vi "obwiednia_DimScreen.vi"() -> ()   [LabVIEW 2012]
uses:
  <vilib>/Analysis/3filter.llb/FIR Filter (DBL).vi
  <vilib>/Analysis/baseanly.llb/Mean (DBL).vi
  <vilib>/addons/Sound and Vibration/Order Analysis/Fault Analysis/SVPO Envelope Detection (1 Ch DBL Array).vi
  <vilib>/Utility/file.llb/Read From Spreadsheet File (DBL).vi
  <vilib>/Utility/file.llb/Write To Spreadsheet File (DBL).vi
  <vilib>/Analysis/4window.llb/Hamming Window (DBL).vi
  <vilib>/Analysis/NI_AALBase.lvlib
  <vilib>/Analysis/NI_AALPro.lvlib
  <vilib>/Analysis/NI_AAL_SigProc.lvlib
  <vilib>/addons/Sound and Vibration/Order Analysis/Fault Analysis/SoundVib_FaultAnalysis.lvlib
  <vilib>/gmath/NI_Gmath.lvlib
  user32.dll
panel:
  out "Maks. indeks":i32
  out "Największy wsp.":dbl
  out "Współczynniki":dbl[](array[numeric])
  out "Odległość":dbl[](array[numeric])
  out "Waveform Graph 3":dbl[](graph)
  in  "Liczenie":bool
  in  "Pomiar":bool
  in  "stop":bool
  out "Signal energy":dbl
  out "Frames":dbl[][](array[numeric])
  out "Przekroczenie progu":bool
  out "Tablica ramek":dbl[](graph)
  out "number of columns":i32
  out "number of rows":i32
  out "Threshold Energy":dbl
  out "Diagram energii":dbl[](graph)
  out "size(s)":i32
  out "sum":dbl
  out "Length":dbl
  out "\"Wygładzona\" energia":dbl[](graph)
  out "max index":dbl
  out "min index":dbl
  out "Wypowiedź":dbl[](graph)
  out "Mowa":waveform(dbl)[](graph)
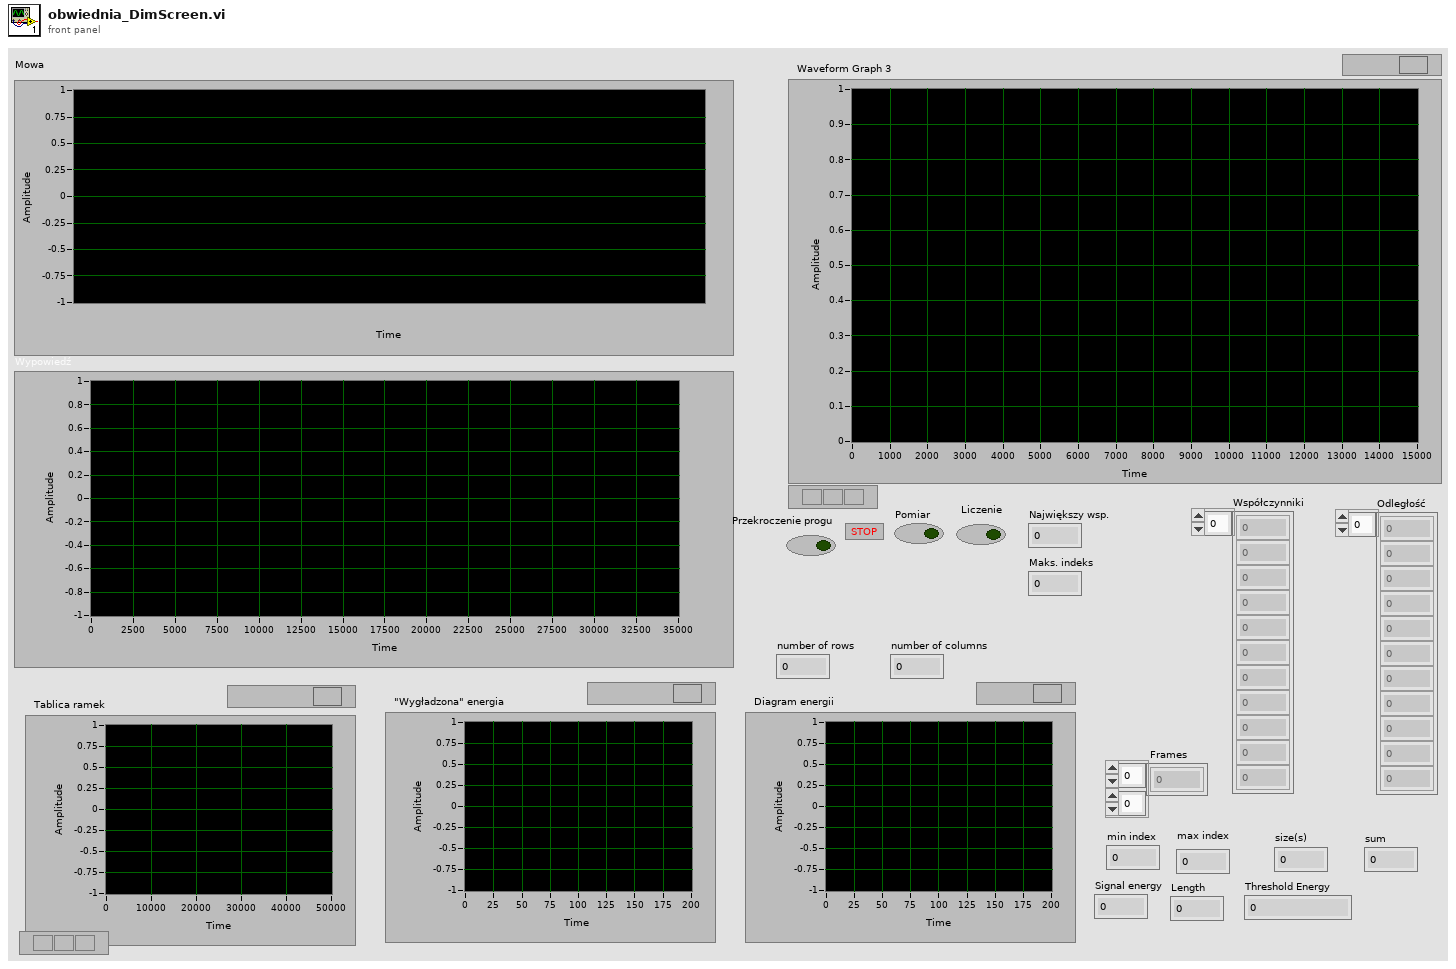
[diagram p1: front panel]
types:
  T1 = enum16{"open", "replace", "create", "open or create", "replace or create", "replace or create with confirmation"}
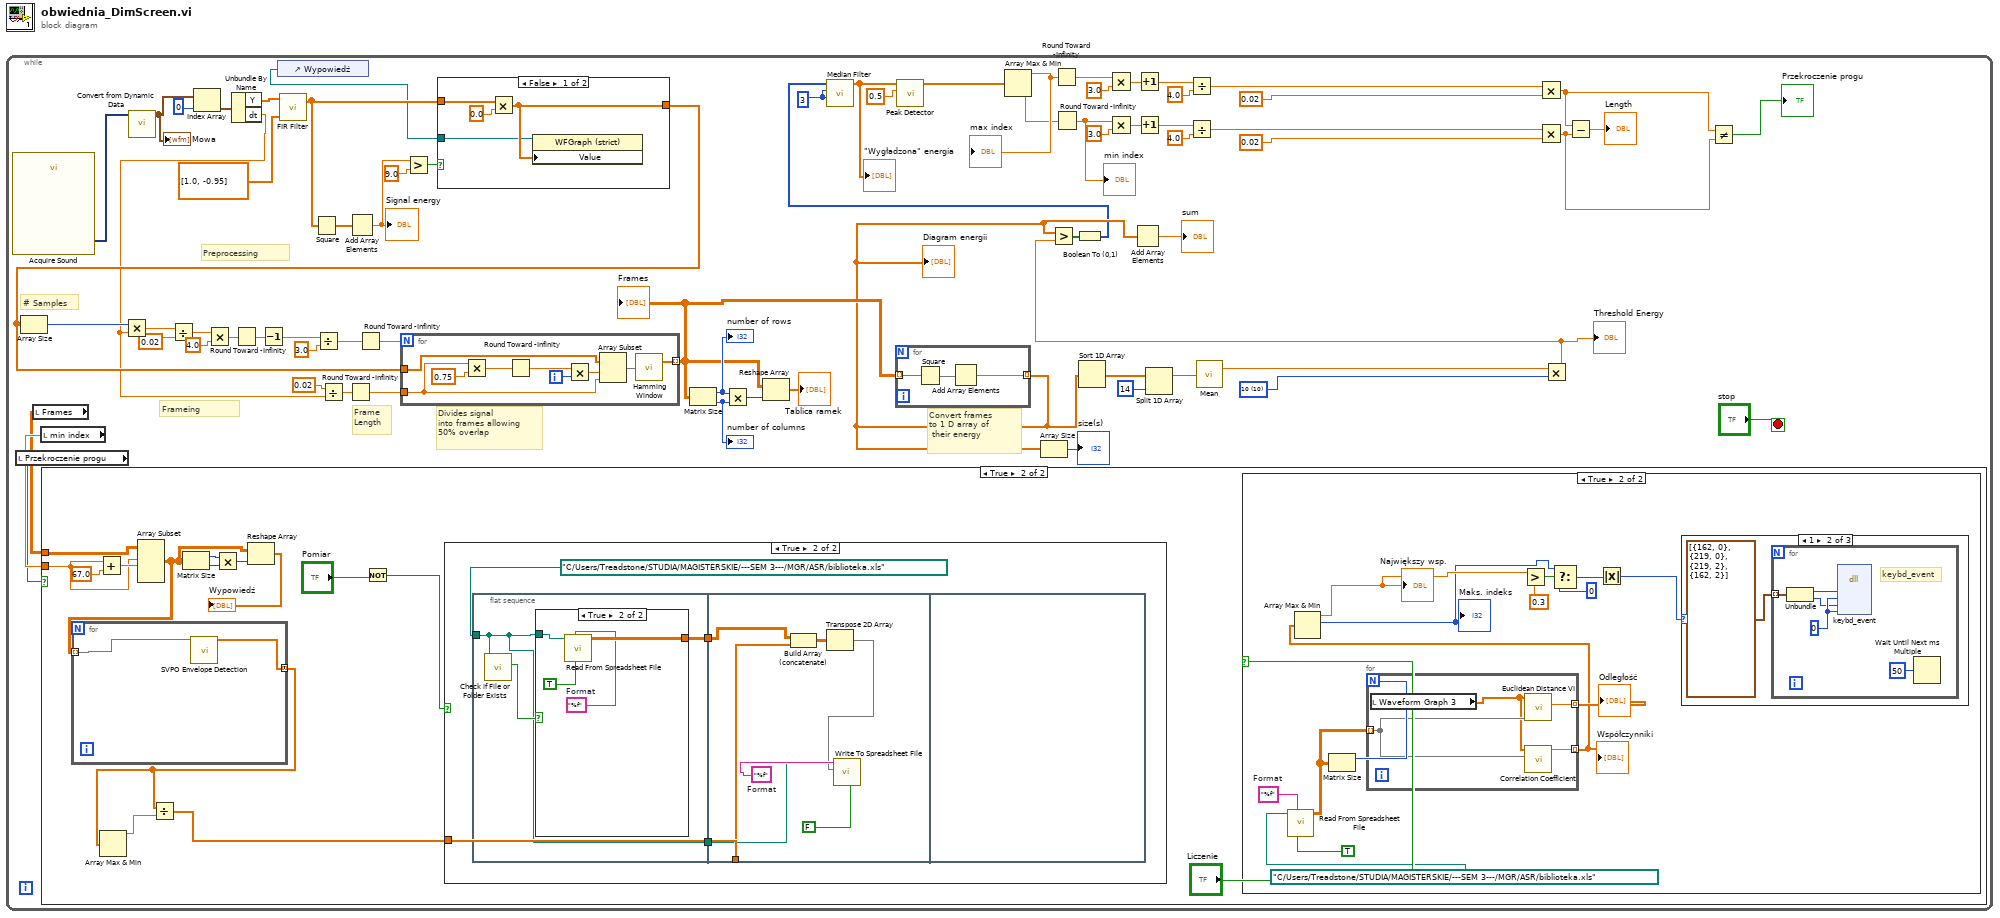
[diagram p0: block diagram]
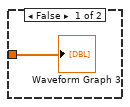
[diagram p3: hidden frame]
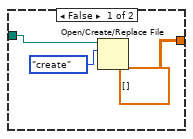
[diagram p4: hidden frame]
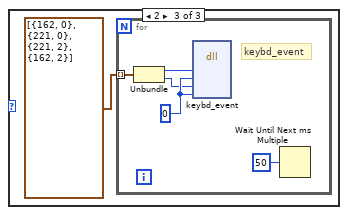
[diagram p7: hidden frame]
diagram:
  n1 = while {
    stop <- "stop" stop-if-true
    w16 = 3 ("right rank")
    w40 = u16 10 items=["5"=5, "6"=6, "7"=7, "9"=9, "10"=10]
    # "Frameing"
    # "Preprocessing"
    # "Convert frames \nto 1 D array of\n their energy"
    # "Divides signal \ninto frames allowing \n50% overlap"
    # "Frame \nLength"
    # "# Samples"
    n2 = call "Acquire Sound"() -> ("Data"=w72:dynamicdata)  [unwired: 18 in, 1 out]
    n3 = local read "Przekroczenie progu"() -> (w2:bool)
    n4 = local read "Frames"() -> (w3:dbl[][])
    n5 = local read "min index"() -> (w4:dbl)
    n6 = case shown="True" w2 {
      tunnel: w4 -> [_ w81]
      tunnel: w3 -> [_ w82]
      frame False {
      }
      frame True {
        n7 = Add(x=w81, y=67.0 ("x")) -> (x+y=w86:dbl)
        n8 = Array Subset(array=w82, index (row)=w81, length (row)=w86) -> (w79:dbl[][])  [unwired: 2 in]
        n9 = for {
          tunnel: w79 -> [w141] mode=indexing
          tunnel: [w140] -> w77 mode=concatenating
          n10 = call-poly <vilib>:"SVPO Envelope Detection.vi"("scaled signal [EU]"=w141) -> ("envelope signal [EU]"=w140:dbl[])  [unwired: 13 in, 1 out]
        }
        n11 = Array Max & Min(array=w77) -> (max value=w78:dbl)  [unwired: 3 out]
        n12 = Divide(x=w77, y=w78) -> (x/y=w75:dbl[])
        n13 = Matrix Size(0:w79) -> (1:w85:i32, 2:w84:i32)
        n14 = Multiply(x=w85, y=w84) -> (x*y=w83:i32)
        n15 = Reshape Array(w79, w83) -> (→"Wypowiedź":dbl[])
        n16 = Not(x="Pomiar") -> (.not. x?=w73:bool)
        n17 = case shown="True" w73 {
          tunnel: w75 -> [w88 w89]
          frame False {
            "Waveform Graph 3" <- w88
          }
          frame True {
            n18 = flat-sequence {
              tunnel: path "C:/Users/Treadstone/STUDIA/MAGISTERSKIE/---SEM 3---/MGR/ASR/biblioteka.xls" ("file path (dialog if empty)") -> [w93]
              tunnel: [w95] -> w92
              tunnel: [w93] -> w91
              tunnel: w92 -> [w103]
              tunnel: w89 -> [w106]
              tunnel: w91 -> [w107]
              frame #0 {
                n19 = call <vilib>:"Check if File or Folder Exists.vi"("path"=w93) -> ("file or folder exists?"=w94:bool)  [unwired: 8 in, 2 out]
                n20 = case shown="True" w94 {
                  tunnel: w93 -> [w98 w102]
                  tunnel: [dbl[][] [] ("all rows") w101] -> w95
                  frame False {
                    n21 = Open/Create/Replace File(file path (use dialog)=w98, operation (0:open)=T1."create") -> ()  [unwired: 4 in, 3 out]
                  }
                  frame True {
                    w100 = "%f"  # Format
                    n22 = call-poly <vilib>:"Read From Spreadsheet File.vi"("transpose (no:F)"=TRUE, "format (%.3f)"=w100, "file path (dialog if empty)"=w102) -> ("all rows"=w101:dbl[][])  [unwired: 4 in, 4 out]
                  }
                }
              }
              frame #1 {
                w109 = "%f"  # Format
                n23 = Build Array (concatenate)(w103, w106) -> (w105:dbl[][])
                n24 = Transpose 2D Array(2D array=w105) -> (transposed array=w104:dbl[][])
                n25 = call-poly <vilib>:"Write To Spreadsheet File.vi"("transpose? (no:F)"=FALSE, "format (%.3f)"=w109, "2D data"=w104, "file path (dialog if empty)"=w107) -> ()  [unwired: 4 in, 1 out]
              }
              frame #2 {
              }
            }
          }
        }
        n26 = case shown="True" "Liczenie" {
          frame False {
          }
          frame True {
            w122 = "%f"  # Format
            n27 = call-poly <vilib>:"Read From Spreadsheet File.vi"("transpose (no:F)"=TRUE, "format (%.3f)"=w122, "file path (dialog if empty)"=path "C:/Users/Treadstone/STUDIA/MAGISTERSKIE/---SEM 3---/MGR/ASR/biblioteka.xls") -> ("all rows"=w117:dbl[][])  [unwired: 4 in, 4 out]
            n28 = Matrix Size(0:w117) -> (1:w120:i32)  [unwired: 1 out]
            n29 = for {
              N: w120 -> [_]
              tunnel: w117 -> [w139] mode=indexing
              tunnel: [w137] -> w119 mode=indexing
              tunnel: [w136] -> w118 mode=indexing
              n30 = local read "Waveform Graph 3"() -> (w138:dbl[])
              n31 = call "Euclidean Distance VI.vi"("Reference"=w139, "Test"=w138) -> ("Dist"=w137:dbl)  [unwired: 9 in]
              n32 = call <vilib>:"Correlation Coefficient.vi"("Y"=w139, "X"=w138) -> ("correlation coefficient r"=w136:dbl)  [unwired: 8 in, 1 out]
            }
            "Odległość" <- w119
            "Współczynniki" <- w118
            n33 = Array Max & Min(array=w118) -> (max value=w112:dbl, max index (indices)=w111:i32)  [unwired: 2 out]
            "Największy wsp." <- w112
            "Maks. indeks" <- w111
            n34 = Greater?(x=w112, y=0.3) -> (0:w116:bool)
            n35 = Select(t=w111, s=w116, f=0) -> (s? t:f=w115:i32)
            n36 = Absolute Value(x=w115) -> (abs(x)=w110:i32)
            n37 = case shown="1" w110 {
              frame 0, Default {
              }
              frame 1 {
                n38 = for {
                  tunnel: cluster{i32, i32}[] [{162, 0}, {219, 0}, {219, 2}, {162, 2}] ("Array") -> [w128] mode=indexing
                  w129 = u32 0 ("dwFlags")
                  # "keybd_event"
                  n39 = Unbundle(w128) -> (w127:i32, w126:i32)
                  n40 = dll-call lib="user32.dll" fn="keybd_event" label="Call Library Function Node"("bVk"=w127, "bScan"=w129, "dwFlags"=w126, "dwExtraInfo"=w129) -> ()  [unwired: 8 in, 2 out]
                  n41 = Wait Until Next ms Multiple(millisecond multiple=u32 50) -> ()  [unwired: 1 out]
                }
              }
              frame 2 {
                n42 = for {
                  tunnel: cluster{i32, i32}[] [{162, 0}, {221, 0}, {221, 2}, {162, 2}] ("Array") -> [w134] mode=indexing
                  w135 = u32 0 ("dwFlags")
                  # "keybd_event"
                  n43 = Unbundle(w134) -> (w133:i32, w132:i32)
                  n44 = dll-call lib="user32.dll" fn="keybd_event" label="Call Library Function Node"("bVk"=w133, "bScan"=w135, "dwFlags"=w132, "dwExtraInfo"=w135) -> ()  [unwired: 8 in, 2 out]
                  n45 = Wait Until Next ms Multiple(millisecond multiple=u32 50) -> ()  [unwired: 1 out]
                }
              }
            }
          }
        }
      }
    }
    n46 = call "Convert from Dynamic Data"("Dynamic Data Type"=w72) -> ("Array of Waveform"=w1:waveform(dbl)[])  [unwired: 3 in]
    "Mowa" <- w1
    n47 = Index Array(array=w1, index=0) -> (element=w62:waveform(dbl))
    n48 = Unbundle By Name(w62) -> ("Y"=w61:dbl[], "dt"=w41:dbl)
    n49 = control-ref of="Wypowiedź"() -> (w5:refnum<vi>)
    n50 = call-poly <vilib>:"FIR Filter.vi"("FIR Coefficients"=dbl[] [1.0, -0.95], "X"=w61) -> ("Filtered X"=w70:dbl[])  [unwired: 2 in, 1 out]
    n51 = Square(x=w70) -> (x^2=w66:dbl[])
    n52 = Divide(x=0.02, y=w41) -> (x/y=w47:dbl)
    n53 = Round Toward -Infinity(1:w47) -> (0:w48:dbl)
    n54 = Add Array Elements(numeric array=w66) -> (sum=w68:dbl)
    "Signal energy" <- w68
    n55 = Greater?(x=w68, y=9.0) -> (0:w69:bool)
    n56 = case shown="False" w69 {
      tunnel: w70 -> [w156 w158]
      tunnel: [w155 w158] -> w42
      tunnel: w5 -> [w154 _]
      frame False {
        n57 = Multiply(x=w156, y=0.0) -> (x*y=w155:dbl[])
        n58 = property class="WFGraph (strict)"(reference=w154, "Value"=w155) -> ()  [unwired: 1 in, 2 out]
      }
      frame True {
      }
    }
    n59 = Array Size(array=w42) -> (size(s)=w60:i32)
    n60 = Multiply(x=w60, y=w41) -> (x*y=w58:dbl)
    n61 = Divide(x=w58, y=0.02) -> (x/y=w54:dbl)
    n62 = Multiply(x=w54, y=4.0) -> (x*y=w53:dbl)
    n63 = Round Toward -Infinity(1:w53) -> (0:w56:dbl)
    n64 = Decrement(x=w56) -> (x-1=w51:dbl)
    n65 = Divide(x=w51, y=3.0) -> (x/y=w50:dbl)
    n66 = Round Toward -Infinity(1:w50) -> (0:w49:dbl)
    n67 = for {
      N: w49 -> [_]
      tunnel: w42 -> [w153]
      tunnel: w48 -> [w150]
      tunnel: [w145] -> w32 mode=indexing
      i -> [w152]
      n68 = Multiply(x=w150, y=0.75 ("x")) -> (x*y=w148:dbl)
      n69 = Round Toward -Infinity(1:w148) -> (0:w147:dbl)
      n70 = Multiply(x=w147, y=w152) -> (x*y=w149:dbl)
      n71 = Array Subset(array=w153, index=w149, length=w150) -> (w146:dbl[])
      n72 = call-poly <vilib>:"Hamming Window.vi"("X"=w146) -> ("Windowed X"=w145:dbl[])  [unwired: 1 out]
    }
    "Frames" <- w32
    n73 = Matrix Size(0:w32) -> (1:w46:i32, 2:w45:i32)
    "number of columns" <- w45
    "number of rows" <- w46
    n74 = Multiply(x=w46, y=w45) -> (x*y=w44:i32)
    n75 = Reshape Array(w32, w44) -> (→"Tablica ramek":dbl[])
    n76 = for {
      tunnel: w32 -> [w144] mode=indexing
      tunnel: [w142] -> w9 mode=indexing
      n77 = Square(x=w144) -> (x^2=w143:dbl[])
      n78 = Add Array Elements(numeric array=w143) -> (sum=w142:dbl)
    }
    "Diagram energii" <- w9
    n79 = Array Size(array=w9) -> (size(s)=→"size(s)":i32)
    n80 = Sort 1D Array(array=w9) -> (sorted array=w36:dbl[])
    n81 = Add Array Elements(numeric array=w9) -> (sum=→"sum":dbl)
    n82 = Split 1D Array(array=w36, index=14) -> (first subarray=w34:dbl[])  [unwired: 1 out]
    n83 = call-poly <vilib>:"Mean.vi"("X"=w34) -> ("mean"=w33:dbl)  [unwired: 1 out]
    n84 = Multiply(x=w33, y=w40) -> (x*y=w39:dbl)
    "Threshold Energy" <- w39
    n85 = Greater?(x=w9, y=w39) -> (0:w38:bool[])
    n86 = Boolean To (0,1)(Boolean=w38) -> (0, 1=w6:i16[])
    n87 = call <vilib>:"Median Filter.vi"("right rank"=w16, "left rank"=w16, "X"=w6) -> ("Filtered X"=w13:dbl[])  [unwired: 7 in, 1 out]
    "\"Wygładzona\" energia" <- w13
    n88 = call <vilib>:"Peak Detector.vi"("threshold"=0.5, "X"=w13) -> ("Locations"=w15:dbl[])  [unwired: 5 in, 4 out]
    n89 = Array Max & Min(array=w15) -> (max value=w17:dbl, min value=w12:dbl)  [unwired: 2 out]
    "max index" <- w17
    n90 = Round Toward -Infinity(1:w17) -> (0:w30:dbl)
    n91 = Round Toward -Infinity(1:w12) -> (0:w11:dbl)
    "min index" <- w11
    n92 = Multiply(x=w30, y=3.0) -> (x*y=w19:dbl)
    n93 = Multiply(x=w11, y=3.0) -> (x*y=w28:dbl)
    n94 = Increment(x=w19) -> (x+1=w20:dbl)
    n95 = Increment(x=w28) -> (x+1=w27:dbl)
    n96 = Divide(x=w20, y=4.0) -> (x/y=w22:dbl)
    n97 = Divide(x=w27, y=4.0) -> (x/y=w25:dbl)
    n98 = Multiply(x=w22, y=0.02) -> (x*y=w8:dbl)
    n99 = Multiply(x=w25, y=0.02) -> (x*y=w7:dbl)
    n100 = Subtract(x=w8, y=w7) -> (x-y=→"Length":dbl)
    n101 = Not Equal?(x=w8, y=w7) -> (x != y?=→"Przekroczenie progu":bool)
  }
